vi "Instruments Abort - PAE.vi"(8 "error in":errorcluster, 11 "PAE Reference in":T1) -> (0 "error out":errorcluster, 3 "PAE Reference Out":T1)   [LabVIEW 2023]
uses:
  <vilib>/niPAEML/Typedefs/Session Handle.ctl
  <vilib>/niPAEML/PAE Reference.lvclass
  <vilib>/niPAEML/PAE Measurement.lvlib
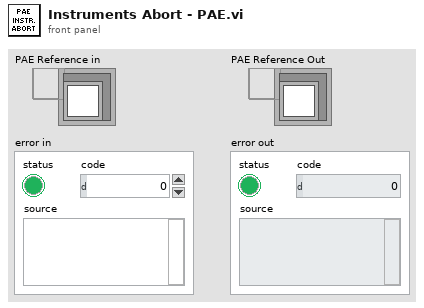
[diagram p1: front panel]
types:
  T1 = typedef "PAE Measurement.lvlib/PAE Reference.lvclass/Session Handle.ctl" = refnum<data-value>
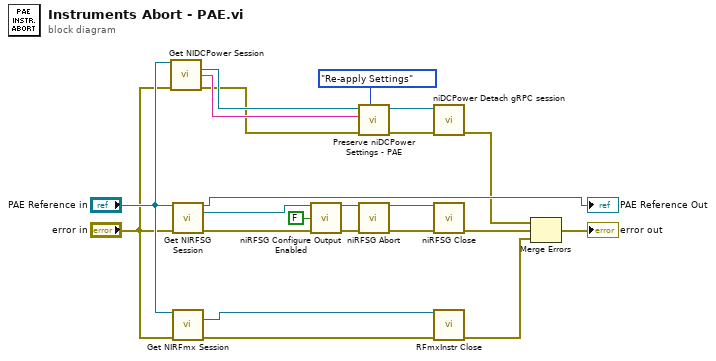
[diagram p0: block diagram]
diagram:
  n1 = call <vilib>:"Get NIDCPower Session.vi"("PAE Reference In"="PAE Reference in", "error in"="error in") -> ("NI DCPower Instrument Handle"=w13:refnum<k15>, "NI DCPower Channel Name"=w12:string, "error out"=w11:errorcluster)  [unwired: 10 in, 1 out]
  n2 = call <vilib>:"Get NIRFSG Session.vi"("PAE Reference In"="PAE Reference in", "error in"="error in") -> ("PAE Reference Out"=→"PAE Reference Out":T1, "NI RFSG Instrument Handle"=w9:refnum<k15>, "error out"=w4:errorcluster)  [unwired: 10 in, 1 out]
  n3 = call <vilib>:"Get NIRFmx Session.vi"("PAE Reference In"="PAE Reference in", "error in"="error in") -> ("NI RFmx Instrument Handle"=w18:refnum<k21>, "error out"=w16:errorcluster)  [unwired: 10 in, 2 out]
  n4 = call <instrlib>:"niRFSG Configure Output Enabled.vi"("instrument handle"=w9, "output enabled"=FALSE ("output enable"), "error in"=w4) -> ("instrument handle out"=w8:refnum<k15>, "error out"=w7:errorcluster)  [unwired: 11 out]
  n5 = call "Preserve niDCPower Settings - PAE.vi"("Action"=enum16{"Reserve Settings", "Re-apply Settings"}."Re-apply Settings", "error in"=w11, "Active Channel"=w12, "Resource Name"=w13) -> ("error out"=w3:errorcluster, "Resource Name"=w1:refnum<k15>)  [unwired: 4 in, 2 out]
  n6 = call <instrlib>:"niRFSG Abort.vi"("instrument handle"=w8, "error in"=w7) -> ("instrument handle out"=w6:refnum<k15>, "error out"=w5:errorcluster)  [unwired: 12 out]
  n7 = call <instrlib>:"niDCPower Detach gRPC session.vi"("error in (no error)"=w3, "instrument handle"=w1) -> ("error out"=w2:errorcluster)  [unwired: 9 in]
  n8 = call <instrlib>:"niRFSG Close.vi"("instrument handle"=w6, "error in"=w5) -> ("error out"=w21:errorcluster)  [unwired: 13 in]
  n9 = call <vilib>:"RFmxInstr Close.vi"("Instrument Handle In"=w18, "error in (no error)"=w16) -> ("error out"=w19:errorcluster)  [unwired: 13 in]
  n10 = Merge Errors(w2, w21, w19) -> (→"error out":errorcluster)
